vi "Write IST bit sense.vi"(8 "error in (no error)":errorcluster, 10 "IST bit sense":bool=TRUE, 11 "RS232 to GPIB ConvBox in":refnum<class "RS-xxx to GPIB ConvBox.lvclass">) -> (0 "error out":errorcluster, 3 "RS232 to GPIB ConvBox out":refnum<class "RS-xxx to GPIB ConvBox.lvclass">)   [LabVIEW 2023, in "Protocols.lvlib" / "RS-xxx to GPIB ConvBox.lvclass"]
uses:
  RS-xxx to GPIB ConvBox.lvclass
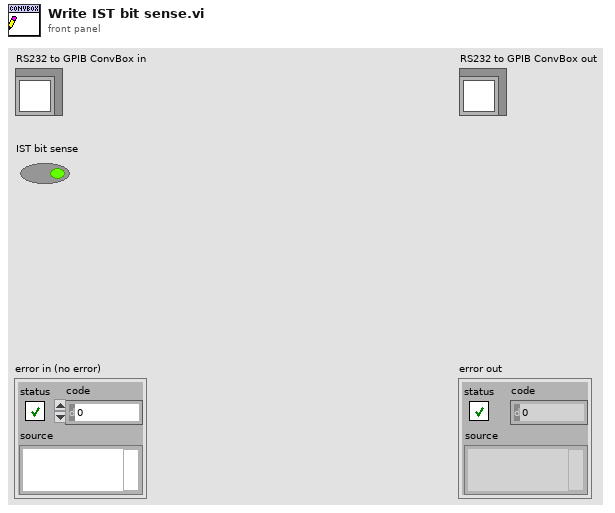
[diagram p1: front panel]
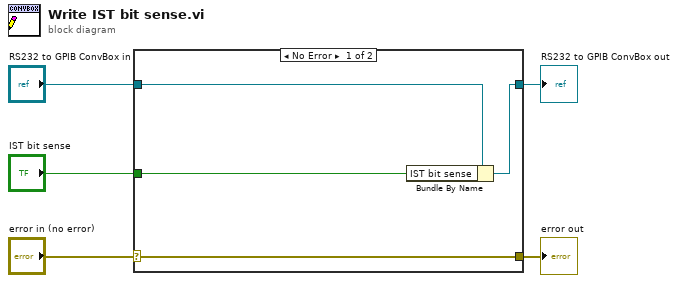
[diagram p0: block diagram]
diagram:
  n1 = case shown="No Error" "error in (no error)" {
    selector: "error in (no error)" -> [w9 w10]
    tunnel: [w9 w10] -> w4
    tunnel: [w7 w11] -> w2
    tunnel: "RS232 to GPIB ConvBox in" -> [w8 w11]
    tunnel: "IST bit sense" -> [w6 _]
    frame No Error {
      n2 = Bundle By Name(cluster=w8, "IST bit sense"=w6) -> (w7:refnum<class "RS-xxx to GPIB ConvBox.lvclass">)
    }
    frame Error {
    }
  }
  "error out" <- w4
  "RS232 to GPIB ConvBox out" <- w2
